vi "Global constant.vi"() -> ()   [LabVIEW 2013]
panel:
  in  "PTC04PSFModule.IPTC04PSFDevice":refnum<k7>
  in  "PSF091206AAMLXModule.IPSF091206AAMLXDevice":refnum<k7>
  out "Stop":bool
  out "MAC ID":string
  out "SN":string
  out "Result":bool
  in  "Model":string
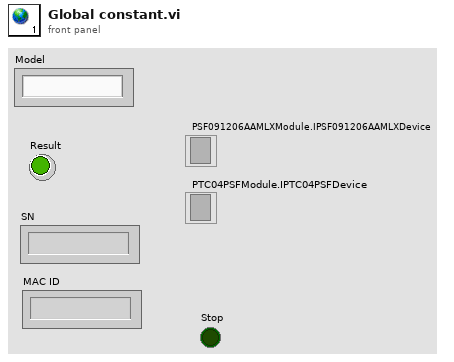
[diagram p1: front panel]
diagram:
